vi "Handle Error.vi"(6 "module reference in":T1, 8 "error in":errorcluster) -> (0 "error out":errorcluster)   [LabVIEW 2017, in "Error Handler.lvlib"]
uses:
  Error Handler.lvlib
  Private TypeDefs/Module Reference.ctl
  Global TypeDefs/Registered Modules.ctl
  Private TypeDefs/Module Queues.ctl
  Private TypeDefs/Message Queue Element.ctl
  Private TypeDefs/Messages.ctl
  Private TypeDefs/Module Notifiers.ctl
  Private TypeDefs/Dummy Notifier.ctl
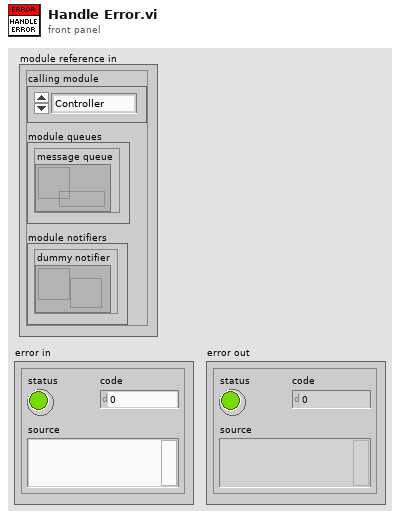
[diagram p1: front panel]
types:
  T1 = typedef "Error Handler.lvlib/Module Reference.ctl" = cluster{"calling module":T2, "module queues":T3, "module notifiers":T4}
  T2 = typedef "Registered Modules.ctl" = enum16{"Controller", "DAQ", "Error Handler", "Game", "myPAM", "WinHost", "Logger"}
  T3 = typedef "Error Handler.lvlib/Module Queues.ctl" = cluster{"message queue":refnum<queue>}
  T4 = typedef "Error Handler.lvlib/Module Notifiers.ctl" = cluster{"dummy notifier":refnum<notifier>}
  T5 = typedef "Error Handler.lvlib/Messages.ctl" = enum16{"handle error", "shutdown"}
  T6 = typedef "Error Handler.lvlib/Message Queue Element.ctl" = cluster{"source":T2, "message":T5, "data":variant}
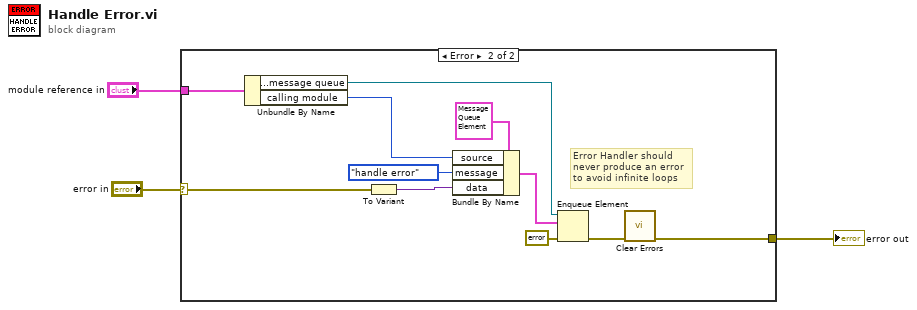
[diagram p0: block diagram]
diagram:
  n1 = case shown="Error" "error in" {
    selector: "error in" -> [w4 w15]
    tunnel: [w4 w13] -> w2
    tunnel: "module reference in" -> [_ w6]
    frame No Error {
    }
    frame Error {
      # "Error Handler should\nnever produce an error\nto avoid infinite loops"
      n2 = Unbundle By Name(w6) -> ("module queues.message queue"=w5:refnum<queue>, "calling module"=w7:T2)
      n3 = To Variant(anything=w15) -> (Variant=w11:variant)
      n4 = Bundle By Name(cluster=T6 {"source"=enum."Controller", "message"=enum."handle error", "data"=variant} ("message queue element"), "source"=w7, "message"=Messages."handle error", "data"=w11) -> (w12:T6)
      n5 = Enqueue Element(queue=w5, element=w12, error in (no error)=errorcluster {"status"=FALSE, "code"=0, "source"=""}) -> (error out=w14:errorcluster)  [unwired: 1 in, 2 out]
      n6 = call <vilib>:"Clear Errors.vi"("error in (no error)"=w14) -> ("error out"=w13:errorcluster)  [unwired: 5 in, 1 out]
    }
  }
  "error out" <- w2
